vi "Convert TDMS.vi"(3 "TXT file to save to":path=path "C:/file.txt", 8 "error in (no error)":errorcluster, 11 "TDMS File to convert from":path=path "C:/test.tdms") -> (0 "error out":errorcluster)   [LabVIEW 2013]
doc: "Reads a TDMS (Technical Data Management Streaming) file."
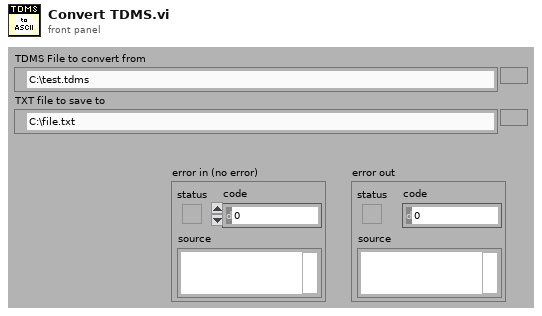
[diagram p1: front panel]
types:
  T1 = enum16{"open", "replace", "create", "open or create", "replace or create", "replace or create with confirmation"}
  T2 = enum16{"open", "open or create", "create or replace", "create", "open (read-only)"}
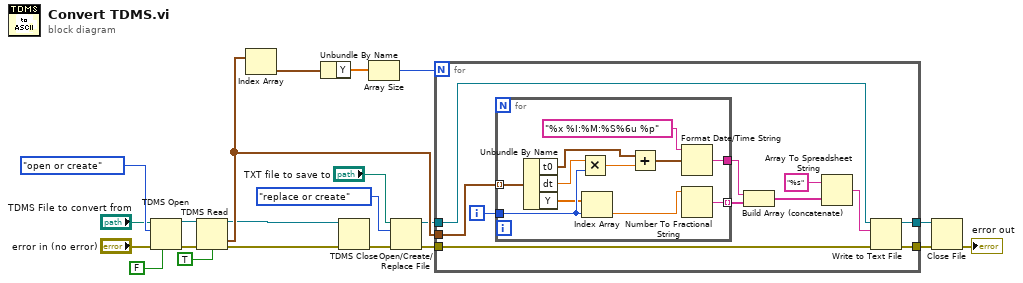
[diagram p0: block diagram]
diagram:
  n1 = TDMS Open(6:FALSE ("disable buffering (T)"), 8:"error in (no error)", 10:T2."open or create" ("operation"), 11:"TDMS File to convert from") -> (0:w19:errorcluster, 3:w20:refnum<k34>)  [unwired: 3 in]
  n2 = TDMS Read(0:w20, 11:w19, 13:TRUE ("파일 순서로 채널 반환? (거짓)")) -> (4:w5:refnum<k34>, 10:w16:waveform(dbl)[], 15:w4:errorcluster)  [unwired: 5 in, 3 out]
  n3 = Index Array(array=w16) -> (element=w15:waveform(dbl))  [unwired: 1 in]
  n4 = Unbundle By Name(w15) -> ("Y"=w14:dbl[])
  n5 = TDMS Close(8:w4, 11:w5) -> (0:w6:errorcluster)  [unwired: 1 out]
  n6 = Array Size(array=w14) -> (size(s)=w8:i32)
  n7 = Open/Create/Replace File(file path (use dialog)="TXT file to save to", error in=w6, operation (0:open)=T1."replace or create") -> (refnum out=w11:refnum<file>, error out=w7:errorcluster)  [unwired: 3 in, 1 out]
  n8 = for {
    N: w8 -> [_]
    tunnel: w16 -> [w32]
    tunnel: w11 -> [w25]
    tunnel: [w24] -> w10
    tunnel: [w23] -> w9
    tunnel: w7 -> [w22]
    i -> [w31]
    n9 = for {
      tunnel: w32 -> [w43] mode=indexing
      tunnel: w31 -> [w39]
      tunnel: [w35] -> w29 mode=indexing
      tunnel: [w34] -> w30
      n10 = Unbundle By Name(w43) -> ("t0"=w40:timestamp, "dt"=w41:dbl, "Y"=w38:dbl[])
      n11 = Multiply(x=w41, y=w39) -> (x*y=w42:dbl)
      n12 = Index Array(array=w38, index=w39) -> (element=w36:dbl)
      n13 = Add(x=w40, y=w42) -> (x+y=w37:timestamp)
      n14 = Format Date/Time String(time format string (%c)="%x %I:%M:%S%6u %p", seconds (now)=w37) -> (date/time string=w34:string)  [unwired: 1 in]
      n15 = Number To Fractional String(number=w36) -> (F-format string=w35:string)  [unwired: 3 in]
    }
    n16 = Build Array (concatenate)(w30, w29) -> (w28:string[])
    n17 = Array To Spreadsheet String(array=w28, 3:"%s" ("format string")) -> (spreadsheet string=w26:string)  [unwired: 1 in]
    n18 = Write to Text File(file (use dialog)=w25, text=w26, error in=w22) -> (refnum out=w23:refnum<file>, error out=w24:errorcluster)  [unwired: 1 in, 1 out]
  }
  n19 = Close File(refnum=w9, error in=w10) -> (error out=→"error out":errorcluster)  [unwired: 1 out]
